vi "良好风格模板VI.vi"() -> ()   [LabVIEW 2017]
panel:
  out "out-of-range":bool
  in  "error in (no error)":errorcluster caption="错误输入（无错误）"
  out "error out":errorcluster caption="错误输出"
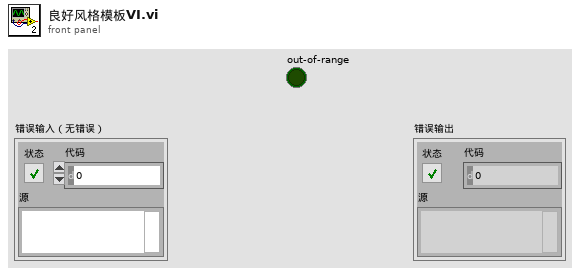
[diagram p1: front panel]
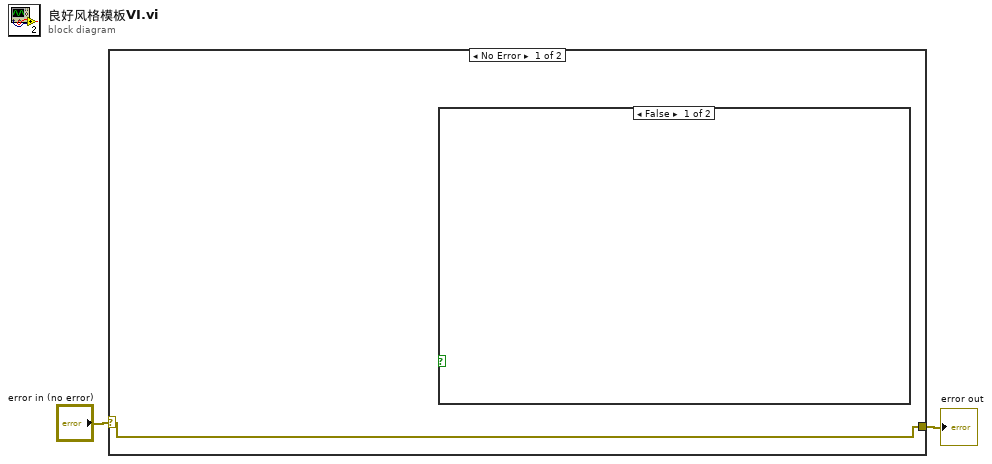
[diagram p0: block diagram]
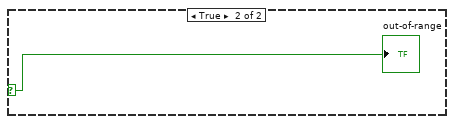
[diagram p2: hidden frame]
diagram:
  n1 = case shown="No Error" "error in (no error)" {
    selector: "error in (no error)" -> [w3 w5]
    tunnel: [w3 w5] -> w1
    frame No Error {
      n2 = case shown="False" {
        selector: _ -> [_ w4]
        frame False {
        }
        frame True {
          "out-of-range" <- w4
        }
      }
    }
    frame Error {
    }
  }
  "error out" <- w1
